vi "ReadAndCheckAttributeType.vi"(8 "error in (no error)":errorcluster, 9 "expected data type":T1, 10 "attribute name":string, 11 "device name":string) -> (0 "error out":errorcluster, 1 "value":u8[](array[numeric]), 2 "dim. y":i32, 3 "dim. x":i32)   [LabVIEW 2014, in "tango.lvlib"]
uses:
  tango.lvlib
  Common VIs/Typedefs/_AttributeDataType_t.ctl
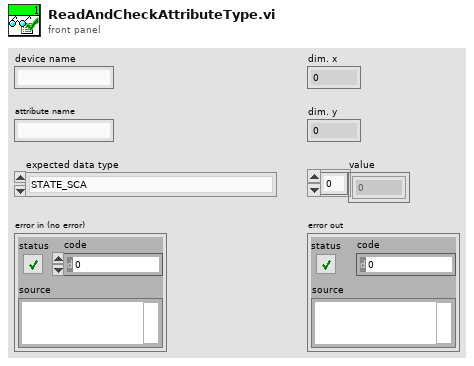
[diagram p1: front panel]
types:
  T1 = typedef "tango.lvlib/_AttributeDataType_t.ctl" = enum16{"STATE_SCA", "STATE_SPE", "STATE_IMG", "STRING_SCA", "STRING_SPE", "STRING_IMG", "BOOL_SCA", "BOOL_SPE", "BOOL_IMG", "UCHAR_SCA", "UCHAR_SPE", "UCHAR_IMG", "SHORT_SCA", "SHORT_SPE", "SHORT_IMG", "USHORT_SCA", "USHORT_SPE", "USHORT_IMG", "LONG_SCA", "LONG_SPE", "LONG_IMG", "ULONG_SCA", "ULONG_SPE", "ULONG_IMG", "LONG64_SCA", "LONG64_SPE", "LONG64_IMG", "ULONG64_SCA", "ULONG64_SPE", "ULONG64_IMG", "FLOAT_SCA", "FLOAT_SPE", "FLOAT_IMG", "DOUBLE_SCA", "DOUBLE_SPE", "DOUBLE_IMG", "UNKNOWN_DATA_TYPE"}
  T2 = cluster{"device name":string, "attribute name":string, "quality value":i16, "quality string":string, "timestamp":dbl, "dim. x":i32, "dim. y":i32, "value":u8[], "error code":i32, "error stack":string[], "data type":u16}[]
  T3 = cluster{"device name":string, "attribute name":string, "quality value":i16, "quality string":string, "timestamp":dbl, "dim. x":i32, "dim. y":i32, "value":u8[], "error code":i32, "error stack":string[], "data type":u16}
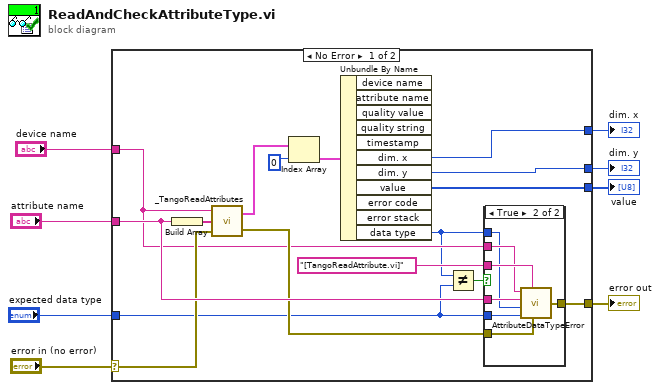
[diagram p0: block diagram]
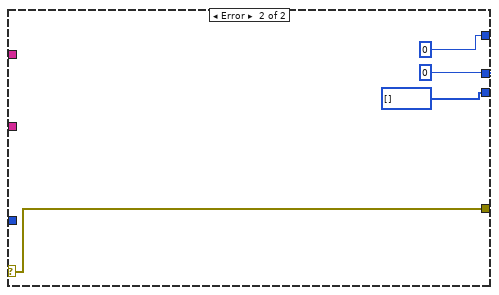
[diagram p3: hidden frame]
diagram:
  n1 = case shown="No Error" "error in (no error)" {
    selector: "error in (no error)" -> [w15 w36]
    tunnel: [w22 0 ("dim. x")] -> w1
    tunnel: [w21 0 ("dim. y")] -> w2
    tunnel: [w20 u8[] [] ("value")] -> w3
    tunnel: [w19 w36] -> w8
    tunnel: "expected data type" -> [w10 _]
    tunnel: "device name" -> [w14 _]
    tunnel: "attribute name" -> [w17 _]
    frame No Error {
      n2 = Build Array(w17) -> (w13:string[])
      n3 = call "_TangoReadAttributes.vi"("error in"=w15, "attribute names"=w13, "device name"=w14) -> ("error out"=w16:errorcluster, "attribute values"=w12:T2)
      n4 = Index Array(array=w12, index=0 ("indice")) -> (element=w23:T3)
      n5 = Unbundle By Name(w23) -> ("dim. x"=w22:i32, "dim. y"=w21:i32, "value"=w20:u8[], "data type"=w11:u16)  [unwired: 7 out]
      n6 = Not Equal?(x=w11, y=w10) -> (x != y?=w9:bool)
      n7 = case shown="True" w9 {
        tunnel: [w25 w32] -> w19
        tunnel: "[TangoReadAttribute.vi]" ("location") -> [_ w31]
        tunnel: w17 -> [_ w30]
        tunnel: w16 -> [w25 w29]
        tunnel: w14 -> [_ w28]
        tunnel: w11 -> [_ w27]
        tunnel: w10 -> [_ w26]
        frame False {
        }
        frame True {
          n8 = call "_AttributeDataTypeError.vi"("error in"=w29, "location"=w31, "user Data Type"=w26, "actual Data Type"=w27, "attribute name"=w30, "device name"=w28) -> ("error out"=w32:errorcluster)
        }
      }
    }
    frame Error {
    }
  }
  "error out" <- w8
  "value" <- w3
  "dim. y" <- w2
  "dim. x" <- w1
